vi "testExample_SetPin.vi"(8 "error in (no error)":errorcluster, 11 "TestCase in":refnum<class "MyTestCase_shido.lvclass">) -> (0 "error out":errorcluster, 3 "TestCase out":refnum<class "MyTestCase_shido.lvclass">)   [LabVIEW 2020, in "MyTestCase_shido.lvclass"]
uses:
  MyTestCase_shido.lvclass
  Implementacion/Simulated/Simulated.lvclass
  <vilib>/addons/_JKI Toolkits/VI Tester/TestCase.llb/TestCase.lvclass
  C:/Program Files/National Instruments/LabVIEW 2020/vi.lib/addons/_JKI Toolkits/VI Tester/TestCase.llb/TestCase.lvclass
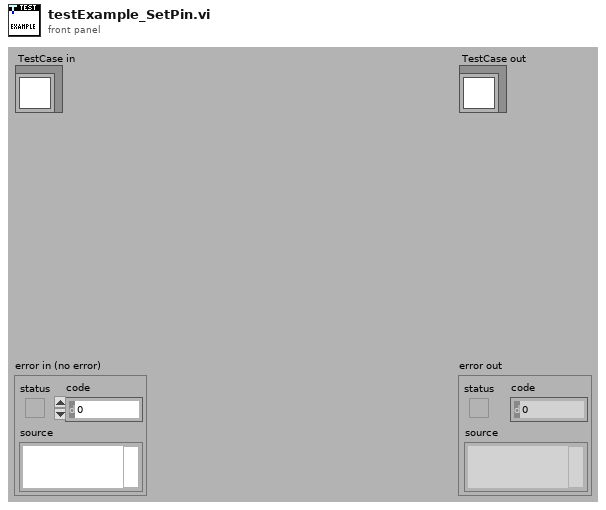
[diagram p1: front panel]
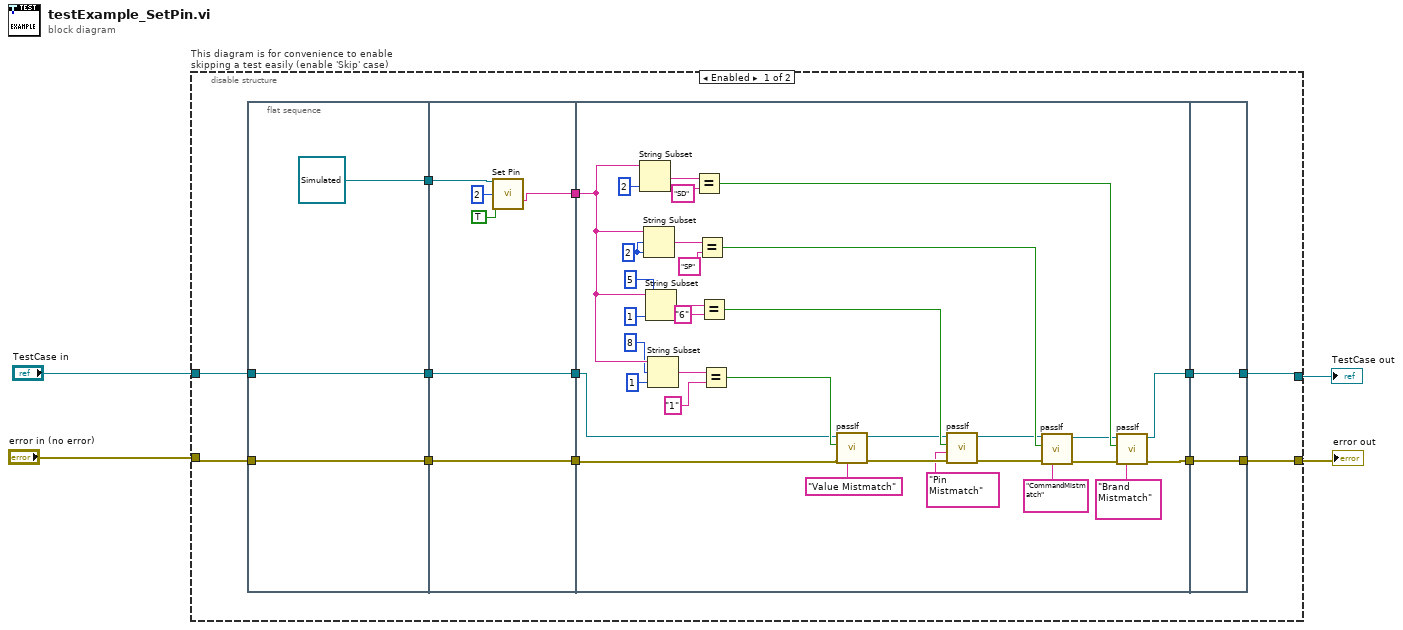
[diagram p0: block diagram]
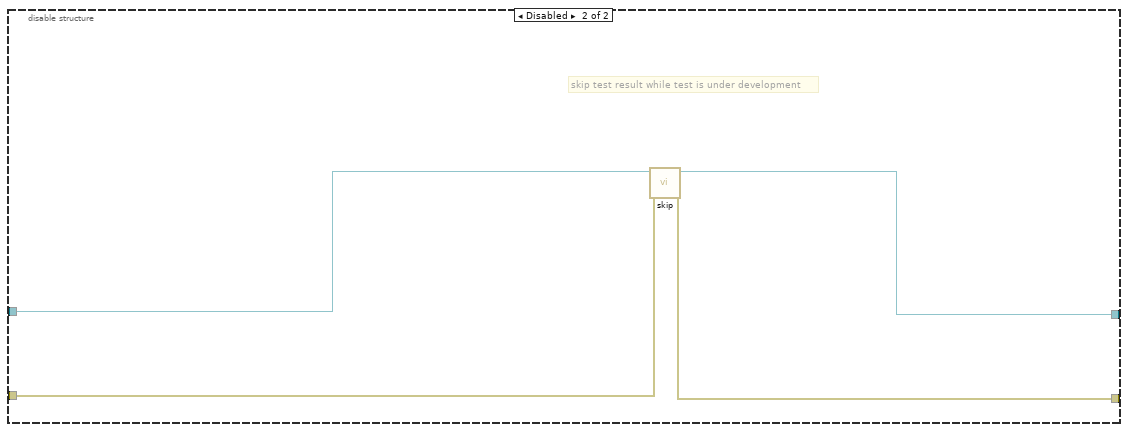
[diagram p2: hidden frame]
diagram:
  n1 = disable-structure "This diagram is for convenience to enable skipping a test easily (enable 'Skip' case)" shown="Enabled" {
    disable-tunnel: "TestCase in" -> [w8 w64]
    disable-tunnel: [w6 w62] -> w1
    disable-tunnel: [w5 w63] -> w3
    disable-tunnel: "error in (no error)" -> [w7 w61]
    frame Enabled {
      n2 = flat-sequence {
        tunnel: w8 -> [w17]
        tunnel: w7 -> [w18]
        tunnel: [refnum<class "Simulated.lvclass"> refnum ("Simulated.lvclass")] -> w16
        tunnel: [w18] -> w15
        tunnel: [w17] -> w14
        tunnel: w16 -> [w22]
        tunnel: [w23] -> w13
        tunnel: w15 -> [w25]
        tunnel: [w25] -> w12
        tunnel: w14 -> [w24]
        tunnel: [w24] -> w11
        tunnel: w13 -> [w48]
        tunnel: w12 -> [w35]
        tunnel: [w43] -> w10
        tunnel: [w30] -> w9
        tunnel: w11 -> [w26]
        tunnel: [w60] -> w5
        tunnel: w10 -> [w60]
        tunnel: w9 -> [w59]
        tunnel: [w59] -> w6
        frame #0 {
        }
        frame #1 {
          n3 = call-dynamic "Set Pin.vi"("Simulated in"=w22, "Pin"=u8 2, "Pin State"=TRUE) -> ("Command send"=w23:string)  [unwired: 9 in, 3 out]
        }
        frame #2 {
          w55 = 2 ("length (rest)")
          n4 = String Subset(string=w48, length (rest)=2 ("length (rest)")) -> (substring=w57:string)  [unwired: 1 in]
          n5 = String Subset(string=w48, offset (0)=w55, length (rest)=w55) -> (substring=w54:string)
          n6 = String Subset(string=w48, offset (0)=5, length (rest)=1 ("length (rest)")) -> (substring=w49:string)
          n7 = String Subset(string=w48, offset (0)=8, length (rest)=1 ("length (rest)")) -> (substring=w45:string)
          n8 = Equal?(x=w57, y="SD") -> (x = y?=w42:bool)
          n9 = Equal?(x=w54, y="SP") -> (x = y?=w39:bool)
          n10 = Equal?(x=w49, y="6") -> (x = y?=w36:bool)
          n11 = Equal?(x=w45, y="1") -> (x = y?=w33:bool)
          n12 = call-dynamic "passIf.vi"("error in (no error)"=w35, "message (\"\")"="Value Mistmatch" ("message (\"\")"), "pass"=w33, "TestCase in"=w26) -> ("error out"=w34:errorcluster, "TestCase out"=w27:refnum<class "MyTestCase_shido.lvclass">)  [unwired: 6 in]
          n13 = call-dynamic "passIf.vi"("error in (no error)"=w34, "message (\"\")"="Pin Mistmatch" ("message (\"\")"), "pass"=w36, "TestCase in"=w27) -> ("error out"=w37:errorcluster, "TestCase out"=w28:refnum<class "MyTestCase_shido.lvclass">)  [unwired: 6 in]
          n14 = call-dynamic "passIf.vi"("error in (no error)"=w37, "message (\"\")"="CommandMistmatch" ("message (\"\")"), "pass"=w39, "TestCase in"=w28) -> ("error out"=w40:errorcluster, "TestCase out"=w29:refnum<class "MyTestCase_shido.lvclass">)  [unwired: 6 in]
          n15 = call-dynamic "passIf.vi"("error in (no error)"=w40, "message (\"\")"="Brand Mistmatch" ("message (\"\")"), "pass"=w42, "TestCase in"=w29) -> ("error out"=w43:errorcluster, "TestCase out"=w30:refnum<class "MyTestCase_shido.lvclass">)  [unwired: 6 in]
        }
        frame #3 {
        }
      }
    }
    frame Disabled {
      # "skip test result while test is under development"
      n16 = call <vilib>:"skip.vi"("error in (no error)"=w61, "TestCase in"=w64) -> ("error out"=w63:errorcluster, "TestCase out"=w62:refnum<class "MyTestCase_shido.lvclass">)  [unwired: 8 in]
    }
  }
  "error out" <- w3
  "TestCase out" <- w1
